vi "XY Graph Save Plot Event.vi"(6 "Delimiter (TAB)":string="\t", 8 "Error In":errorcluster, 11 "AliGator Save Plot Data":T1) -> (0 "Error Out":errorcluster, 1 "Message":string, 2 "File Path":path, 3 "Plot Name":string, 4 "Saved Plot Index":i32, 5 "Graph Caption":string)   [LabVIEW 2021, in "XY Graph Add-Ons.lvlib"]
uses:
  XY Graph Add-Ons.lvlib
  <vilib>/Utility/miscctls.llb/LVPoint32TypeDef.ctl
  Get Plot at Mouse Click (XY Graph)/Get Plot at Mouse Click [AAC].vi
  Graphs.lvlib
  XY Graph Save Plot Data.ctl
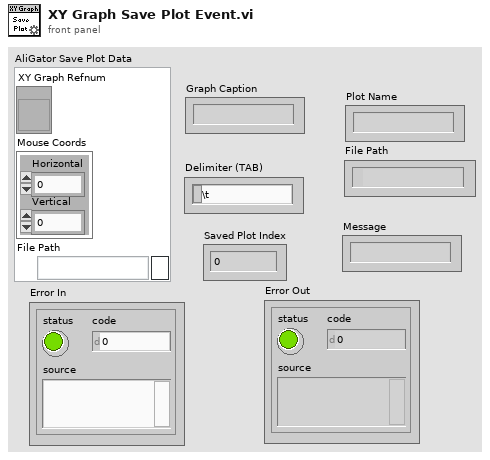
[diagram p1: front panel]
types:
  T1 = typedef "XY Graph Add-Ons.lvlib/XY Graph Save Plot Data.ctl" = cluster{"XY Graph Refnum":refnum<vi>, "Mouse Coords":T2, "File Path":path}
  T2 = typedef "LVPoint32TypeDef.ctl" = cluster{"Horizontal":i32, "Vertical":i32}
  T3 = typedef "XY Graph Add-Ons.lvlib/XY Graph Refnum.ctl" = refnum<vi>
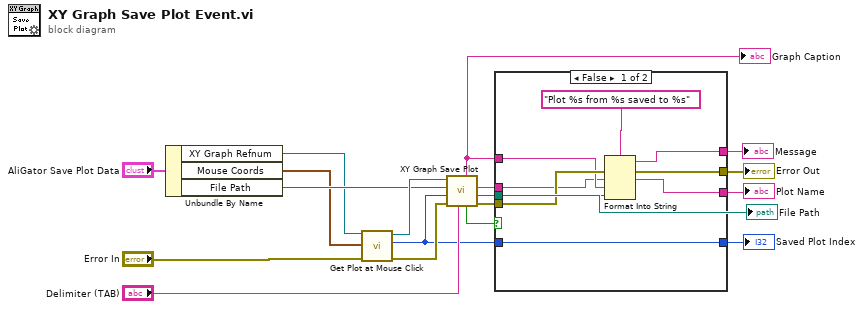
[diagram p0: block diagram]
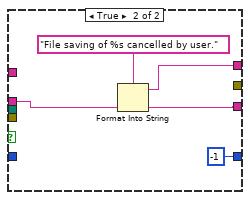
[diagram p2: hidden frame]
diagram:
  n1 = Unbundle By Name("AliGator Save Plot Data") -> ("XY Graph Refnum"=w2:refnum<vi>, "Mouse Coords"=w1:T2, "File Path"=w3:path)
  n2 = call-poly "Get Plot at Mouse Click.vi"("error in (no error)"="Error In", "Mouse Click Coordinates"=w1, "XYGraph Ref"=w2) -> ("error out"=w16:errorcluster, "Plot at Coordinates"=w7:i32, "XYGraph Ref"=w18:T3)  [unwired: 2 in, 4 out]
  n3 = call "XY Graph Save Plot.vi"("Delimiter (TAB)"="Delimiter (TAB)", "Error In"=w16, "Plot Index (-1: last plot)"=w7, "File Path (empty: dialog)"=w3, "XYGraph Ref"=w18) -> ("Error Out"=w14:errorcluster, "File Path"=w13:path, "Plot Name"=w9:string, "Cancelled"=w8:bool, "Graph Name"=w10:string)  [unwired: 1 in, 1 out]
  "Graph Caption" <- w10
  "File Path" <- w13
  n4 = case shown="False" w8 {
    tunnel: w14 -> [w25 _]
    tunnel: w13 -> [w24 _]
    tunnel: [w23 _] -> w12
    tunnel: [w22 w27] -> w11
    tunnel: w10 -> [w21 _]
    tunnel: w9 -> [w19 w28]
    tunnel: w7 -> [w20 _]
    tunnel: [w20 -1 ("Plot at Coordinates")] -> w6
    tunnel: [w19 w28] -> w5
    frame False {
      n5 = Format Into String(format string="Plot %s from %s saved to %s", error in=w25, w19, w21, w24) -> (resulting string=w22:string, error out=w23:errorcluster)  [unwired: 1 in]
    }
    frame True {
      n6 = Format Into String(format string="File saving of %s cancelled by user.", w28) -> (resulting string=w27:string)  [unwired: 2 in, 1 out]
    }
  }
  "Error Out" <- w12
  "Saved Plot Index" <- w6
  "Plot Name" <- w5
  "Message" <- w11
